vi "_demo.vi"() -> ()   [LabVIEW 2019]
uses:
  <userlib>/MicroPython/VIs/uPythonX/uPythonX.xctl
  <userlib>/MicroPython/VIs/PythonGenerator/_subs/utime_sleep_sec.vi
  <userlib>/MicroPython/VIs/PythonGenerator/_subs/utime_sleep_ms.vi
panel:
  out "Pot 2":T1(xcontrol)={"VISA Refnum in"="ASRL44::INSTR", "Python Code"="'''\nhttp://wiki.seeedstudio.com/Grove-Button/\n\nconnections: \nGround  - GND \nPower    - 3V3 \nNC\nSignal -  pin Y9\n'''\n\nfrom pyb import Pin\n\nclass GroveButton(object):\n    def __init__(self, pin):\n         self.button = Pin(pin,Pin.IN)\n\n    def value(self):\n        return self.button.value()\n        \nbutton = GroveButton('Y9')\nbutton.value()"}
  out "Pot":T1(xcontrol)={"VISA Refnum in"="ASRL44::INSTR", "Python Code"="'''\nhttp://wiki.seeedstudio.com/Grove-Button/\n\nconnections: \nGround  - GND \nPower    - 3V3 \nNC\nSignal -  pin Y9\n'''\n\nfrom pyb import Pin\n\nclass GroveButton(object):\n    def __init__(self, pin):\n         self.button = Pin(pin,Pin.IN)\n\n    def value(self):\n        return self.button.value()\n        \nbutton = GroveButton('Y9')\nbutton.value()"}
  out "Button":T1(xcontrol)={"VISA Refnum in"="ASRL44::INSTR", "Python Code"="'''\nhttp://wiki.seeedstudio.com/Grove-Button/\n\nconnections: \nGround  - GND \nPower    - 3V3 \nNC\nSignal -  pin Y9\n'''\n\nfrom pyb import Pin\n\nclass GroveButton(object):\n    def __init__(self, pin):\n         self.button = Pin(pin,Pin.IN)\n\n    def value(self):\n        return self.button.value()\n        \nbutton = GroveButton('Y9')\nbutton.value()"}
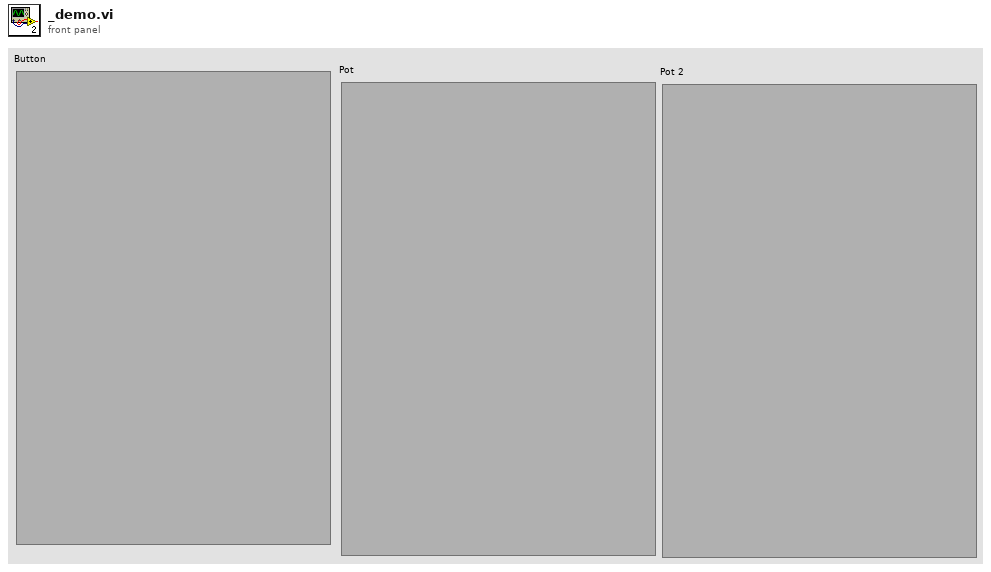
[diagram p1: front panel]
types:
  T1 = cluster{"VISA Refnum in":refnum<visa-resource-name>, "Python Code":string}
  T2 = typedef "uPythonX.xctl/PythonData.ctl" = cluster{"Port":refnum<visa-resource-name>, "All Code":string}
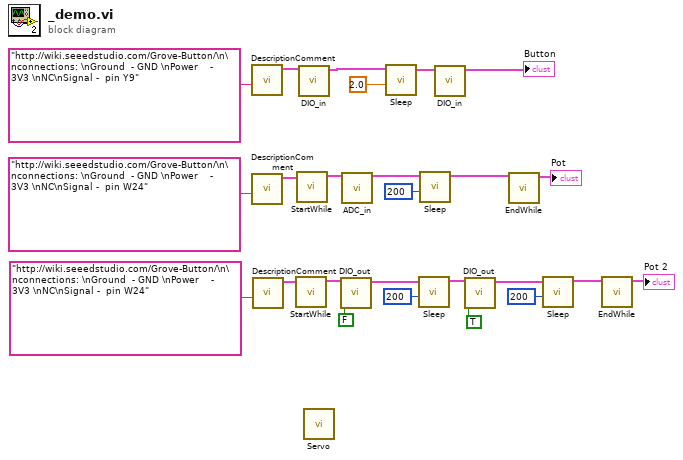
[diagram p0: block diagram]
diagram:
  n1 = call <userlib>:"DescriptionComment.vi"("Description"="http://wiki.seeedstudio.com/Grove-Button/\n\nconnections: \nGround  - GND \nPower    - 3V3 \nNC\nSignal -  pin Y9") -> ("Data Out"=w24:T2)  [unwired: 10 in]
  n2 = call <userlib>:"DescriptionComment.vi"("Description"="http://wiki.seeedstudio.com/Grove-Button/\n\nconnections: \nGround  - GND \nPower    - 3V3 \nNC\nSignal -  pin W24") -> ("Data Out"=w20:T2)  [unwired: 10 in]
  n3 = call <userlib>:"DescriptionComment.vi"("Description"="http://wiki.seeedstudio.com/Grove-Button/\n\nconnections: \nGround  - GND \nPower    - 3V3 \nNC\nSignal -  pin W24") -> ("Data Out"=w10:T2)  [unwired: 10 in]
  n4 = call <userlib>:"StartWhile.vi"("Data In"=w10) -> ("Data Out"=w8:T2)  [unwired: 10 in]
  n5 = call <userlib>:"StartWhile.vi"("Data In"=w20) -> ("Data Out"=w21:T2)  [unwired: 10 in]
  n6 = call <userlib>:"DIO_in.vi"("Data In"=w24) -> ("Data Out"=w18:T2)  [unwired: 10 in]
  n7 = call <userlib>:"Servo.vi"() -> ()  [unwired: 11 in, 1 out]
  n8 = call <userlib>:"DIO_out.vi"("State"=FALSE, "Data In"=w8) -> ("Data Out"=w7:T2)  [unwired: 9 in]
  n9 = call <userlib>:"ADC_in.vi"("Data In"=w21) -> ("Data Out"=w14:T2)  [unwired: 10 in]
  n10 = call-poly <userlib>:"Sleep.vi"("wait (s)"=2.0, "Data In"=w18) -> ("Data Out"=w17:T2)  [unwired: 9 in]
  n11 = call-poly <userlib>:"Sleep.vi"("wait (ms)"=u32 200, "Data In"=w7) -> ("Data Out"=w4:T2)  [unwired: 9 in]
  n12 = call-poly <userlib>:"Sleep.vi"("wait (ms)"=u32 200, "Data In"=w14) -> ("Data Out"=w15:T2)  [unwired: 9 in]
  n13 = call <userlib>:"DIO_in.vi"("Data In"=w17) -> ("Data Out"=→"Button":T2)  [unwired: 10 in]
  n14 = call <userlib>:"DIO_out.vi"("State"=TRUE, "Data In"=w4) -> ("Data Out"=w6:T2)  [unwired: 9 in]
  n15 = call <userlib>:"EndWhile.vi"("Data In"=w15) -> ("Data Out"=→"Pot":T2)  [unwired: 10 in]
  n16 = call-poly <userlib>:"Sleep.vi"("wait (ms)"=u32 200, "Data In"=w6) -> ("Data Out"=w3:T2)  [unwired: 9 in]
  n17 = call <userlib>:"EndWhile.vi"("Data In"=w3) -> ("Data Out"=→"Pot 2":T2)  [unwired: 10 in]
